vi "AckNack.vi"(8 "error in (no error)":errorcluster, 9 "Original TCP Payload":T2, 10 "Result":T1, 11 "TCPMessaging in":refnum<class "TCPMessaging.lvclass">) -> (0 "error out":errorcluster, 3 "TCPMessaging out":refnum<class "TCPMessaging.lvclass">)   [LabVIEW 2020]
uses:
  TCPMessaging.lvclass/TCPMessaging.ctl
  proto/AckNackResult/Enumeration.ctl
  proto/AckNackResult/AckNackResult.lvlib
  proto/TcpAckNack/Data.ctl
  proto/TcpAckNack/TcpAckNack.lvlib
  TCPMessaging.lvclass
  proto/TcpPayload/Data.ctl
  proto/TcpPayload/TcpPayload.lvlib
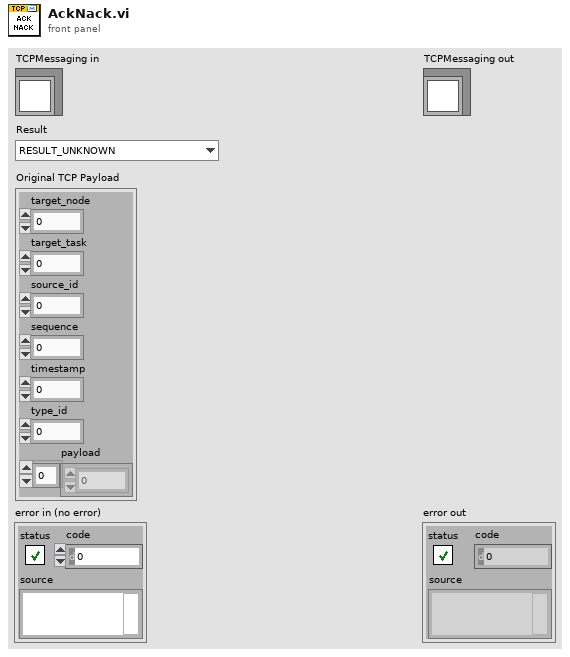
[diagram p1: front panel]
types:
  T1 = typedef "AckNackResult.lvlib/Enumeration.ctl" = enum16{"RESULT_UNKNOWN", "RESULT_INVALIDTARGET", "RESULT_INVALIDTASK", "RESULT_DISALLOWED", "RESULT_OUTOFSEQUENCE", "RESULT_EXPIRED", "RESULT_UNEXPECTED_TYPE", "RESULT_PAYLOAD_ERROR", "RESULT_RECEIVED"}
  T2 = typedef "TcpPayload.lvlib/Data.ctl" = cluster{"target_node":u32, "target_task":u32, "source_id":u32, "sequence":u32, "timestamp":u64, "type_id":u32, "payload":u8[]}
  T3 = typedef "TcpAckNack.lvlib/Data.ctl" = cluster{"target_node":u32, "target_task":u32, "sequence":u32, "timestamp":u64, "type_id":u32, "result":T1}
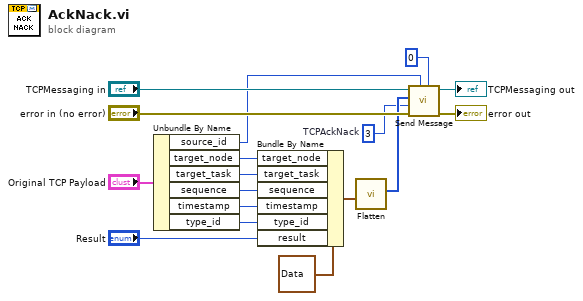
[diagram p0: block diagram]
diagram:
  w3 = u32 3  # TCPAckNack
  n1 = Unbundle By Name("Original TCP Payload") -> ("source_id"=w4:u32, "target_node"=w13:u32, "target_task"=w12:u32, "sequence"=w11:u32, "timestamp"=w10:u64, "type_id"=w7:u32)
  n2 = Bundle By Name(cluster=T3 {"target_node"=0, "target_task"=0, "sequence"=0, "timestamp"=0, "type_id"=0, "result"=enum."RESULT_UNKNOWN"} ("TcpNack"), "target_node"=w13, "target_task"=w12, "sequence"=w11, "timestamp"=w10, "type_id"=w7, "result"="Result") -> (w9:T3)
  n3 = call "Flatten.vi"("Data"=w9) -> ("Buffer"=w5:u8[])  [unwired: 9 in, 1 out]
  n4 = call "Send Message.vi"("Target Task"=u32 0, "Target Node"=w4, "error in (no error)"="error in (no error)", "Type ID"=w3, "Payload"=w5, "TCPMessaging in"="TCPMessaging in") -> ("error out"=→"error out":errorcluster, "TCPMessaging out"=→"TCPMessaging out":refnum<class "TCPMessaging.lvclass">)  [unwired: 4 in]
